vi "Helper SubVI - Image Fusion.vi"(5 "wavelet":u16(ring)=13 items=["Haar"=13, "bior2_2"=16, "bior4_4 (FBI)"=25], 6 "fusion method":cluster{"approximation":u16, "detail":u16}={"approximation"=2, "detail"=0} {"detail" items=["Max", "Min", "Mean", "Image 1", "Image 2"]; "approximation" items=["Max", "Min", "Mean", "Image 1", "Image 2"]}, 7 "extension":u16(ring)=1 items=["zero padding", "symmetric", "periodic"], 8 "error in (no error)":errorcluster, 9 "level":i32=-1, 10 "Image 2":i32[][](array[numeric]), 11 "Image 1":i32[][](array[numeric])) -> (0 "error out":errorcluster, 3 "Fusion Image":i32[][](array[numeric]))   [LabVIEW 2023]
doc: "Computes the detail and approximation coefficients of two images using the WA Discrete Wavelet Transform VI, merges the resulting coefficients, and computes the fusion image using the WA Inverse Discrete Wavelet Transform VI."
uses:
  <vilib>/addons/Wavelet Analysis/discrete wavelet transform.llb/WA 2D Integer Wavelet Transform.vi
  <vilib>/addons/Wavelet Analysis/discrete wavelet transform.llb/WA Inverse 2D Integer Wavelet Transform.vi
  <vilib>/addons/_Advanced Signal Processing/NI_AdvSigProcWA.lvlib
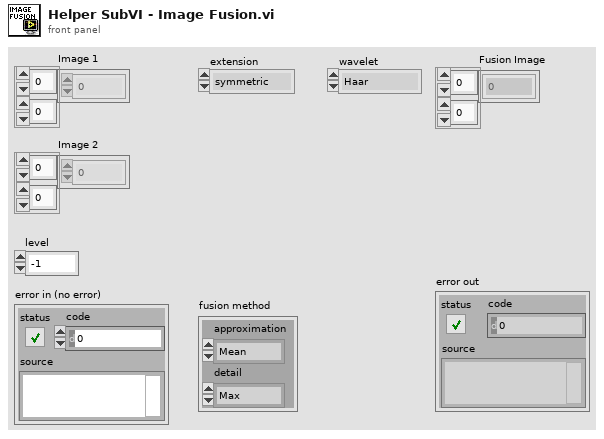
[diagram p1: front panel]
types:
  T1 = cluster{"low_low":i32[][], "low_high":i32[][], "high_low":i32[][], "high_high":i32[][]}[]
  T2 = cluster{"low_low":i32[][], "low_high":i32[][], "high_low":i32[][], "high_high":i32[][]}
  T3 = cluster{"low_low":i32[][], "Fusion Coef":i32[][], "Fusion Coef":i32[][], "Fusion Coef":i32[][]}
  T4 = cluster{"low_low":i32[][], "Fusion Coef":i32[][], "Fusion Coef":i32[][], "Fusion Coef":i32[][]}[]
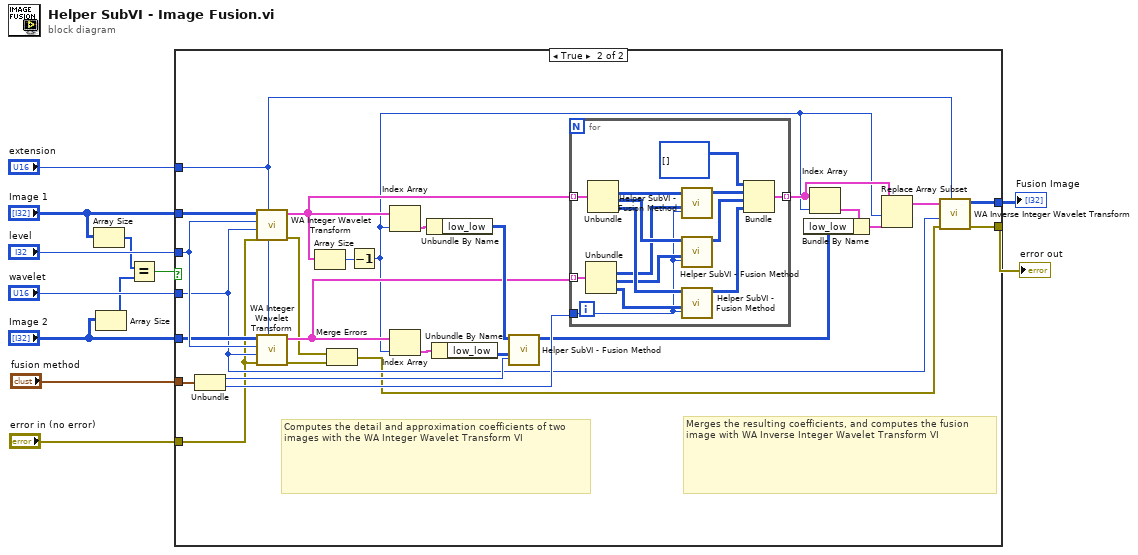
[diagram p0: block diagram]
diagram:
  n1 = Array Size(array="Image 1") -> (size(s)=w7:i32[])
  n2 = Array Size(array="Image 2") -> (size(s)=w6:i32[])
  n3 = Equal?(x=w7, y=w6) -> (x = y?=w5:bool)
  n4 = case shown="True" w5 {
    tunnel: "extension" -> [_ w18]
    tunnel: "level" -> [_ w40]
    tunnel: "wavelet" -> [_ w22]
    tunnel: "Image 1" -> [_ w21]
    tunnel: "Image 2" -> [_ w39]
    tunnel: "fusion method" -> [_ w38]
    tunnel: [_ w20] -> w3
    tunnel: [w13 w19] -> w2
    tunnel: "error in (no error)" -> [w13 w17]
    frame False {
    }
    frame True {
      # "Merges the resulting coefficients, and computes the fusion image with WA Inverse Integer Wavelet Transform VI"
      # "Computes the detail and approximation coefficients of two images with the WA Integer Wavelet Transform VI"
      n5 = Unbundle(w38) -> ("approximation"=w32:u16, "detail"=w29:u16)
      n6 = call-poly <vilib>:"WA Integer Wavelet Transform.vi"("extension"=w18, "error in (no error)"=w17, "wavelet"=w22, "levels"=w40, "signal"=w21) -> ("error out"=w16:errorcluster, "IWT coef"=w31:T1)  [unwired: 5 out]
      n7 = call-poly <vilib>:"WA Integer Wavelet Transform.vi"("extension"=w18, "error in (no error)"=w17, "wavelet"=w22, "levels"=w40, "signal"=w39) -> ("error out"=w15:errorcluster, "IWT coef"=w30:T1)  [unwired: 5 out]
      n8 = Array Size(array=w31) -> (size(s)=w37:i32)
      n9 = Merge Errors(w16, w15) -> (w14:errorcluster)
      n10 = Decrement(x=w37) -> (x-1=w24:i32)
      n11 = Index Array(array=w31, index=w24) -> (element=w36:T2)
      n12 = Index Array(array=w30, index=w24) -> (element=w35:T2)
      n13 = Unbundle By Name(w36) -> ("low_low"=w34:i32[][])
      n14 = Unbundle By Name(w35) -> ("low_low"=w33:i32[][])
      n15 = call "Helper SubVI - Fusion Method.vi"("method"=w32, "Coef 2"=w33, "Coef 1"=w34) -> ("Fusion Coef"=w27:i32[][])  [unwired: 8 in]
      n16 = for {
        tunnel: w31 -> [w54] mode=indexing
        tunnel: w30 -> [w53] mode=indexing
        tunnel: w29 -> [w46]
        tunnel: [w42] -> w26 mode=indexing
        n17 = Unbundle(w53) -> ("low_high"=w49:i32[][], "high_low"=w48:i32[][], "high_high"=w47:i32[][])  [unwired: 1 out]
        n18 = Unbundle(w54) -> ("low_high"=w52:i32[][], "high_low"=w51:i32[][], "high_high"=w50:i32[][])  [unwired: 1 out]
        n19 = call "Helper SubVI - Fusion Method.vi"("method"=w46, "Coef 2"=w49, "Coef 1"=w52) -> ("Fusion Coef"=w45:i32[][])  [unwired: 8 in]
        n20 = call "Helper SubVI - Fusion Method.vi"("method"=w46, "Coef 2"=w48, "Coef 1"=w51) -> ("Fusion Coef"=w44:i32[][])  [unwired: 8 in]
        n21 = call "Helper SubVI - Fusion Method.vi"("method"=w46, "Coef 2"=w47, "Coef 1"=w50) -> ("Fusion Coef"=w43:i32[][])  [unwired: 8 in]
        n22 = Bundle("low_low"=i32[][] [], "Fusion Coef"=w45, "Fusion Coef"=w44, "Fusion Coef"=w43) -> (w42:T3)  [unwired: 1 out]
      }
      n23 = Index Array(array=w26, index=w24) -> (element=w28:T3)
      n24 = Bundle By Name(cluster=w28, "low_low"=w27) -> (w25:T3)
      n25 = Replace Array Subset(array=w26, new element=w25, index=w24) -> (w23:T4)
      n26 = call-poly <vilib>:"WA Inverse Integer Wavelet Transform.vi"("extension"=w18, "error in (no error)"=w14, "wavelet"=w22, "IWT coef"=w23) -> ("error out"=w19:errorcluster, "signal"=w20:i32[][])  [unwired: 6 out]
    }
  }
  "Fusion Image" <- w3
  "error out" <- w2
